vi "英维克通讯.vi"() -> ()   [LabVIEW 2016, in "环境动力监测库.lvlib" / "空调库.lvlib"]
uses:
  <vilib>/Plasmionique/MB Master/MB_Master/MB_Master.lvclass
  <vilib>/Plasmionique/MB Master/MB Master.lvlib
panel:
  out "遥控开关机状态":bool
  out "系统参数":T1
  out "告警状态":T2
  out "传感器状态":T3
  out "运行状态":T4
  out "遥控参数":u16[](array[numeric])
  out "系统参数":u16[](array[numeric])
  out "告警状态":u16[](array[numeric])
  out "传感器状态":u16[](array[numeric])
  out "运行状态":u16[](array[numeric])
  in  "读取数据":bool
  in  "释放串口":bool
  in  "打开串口":bool
  out "通讯状态":bool
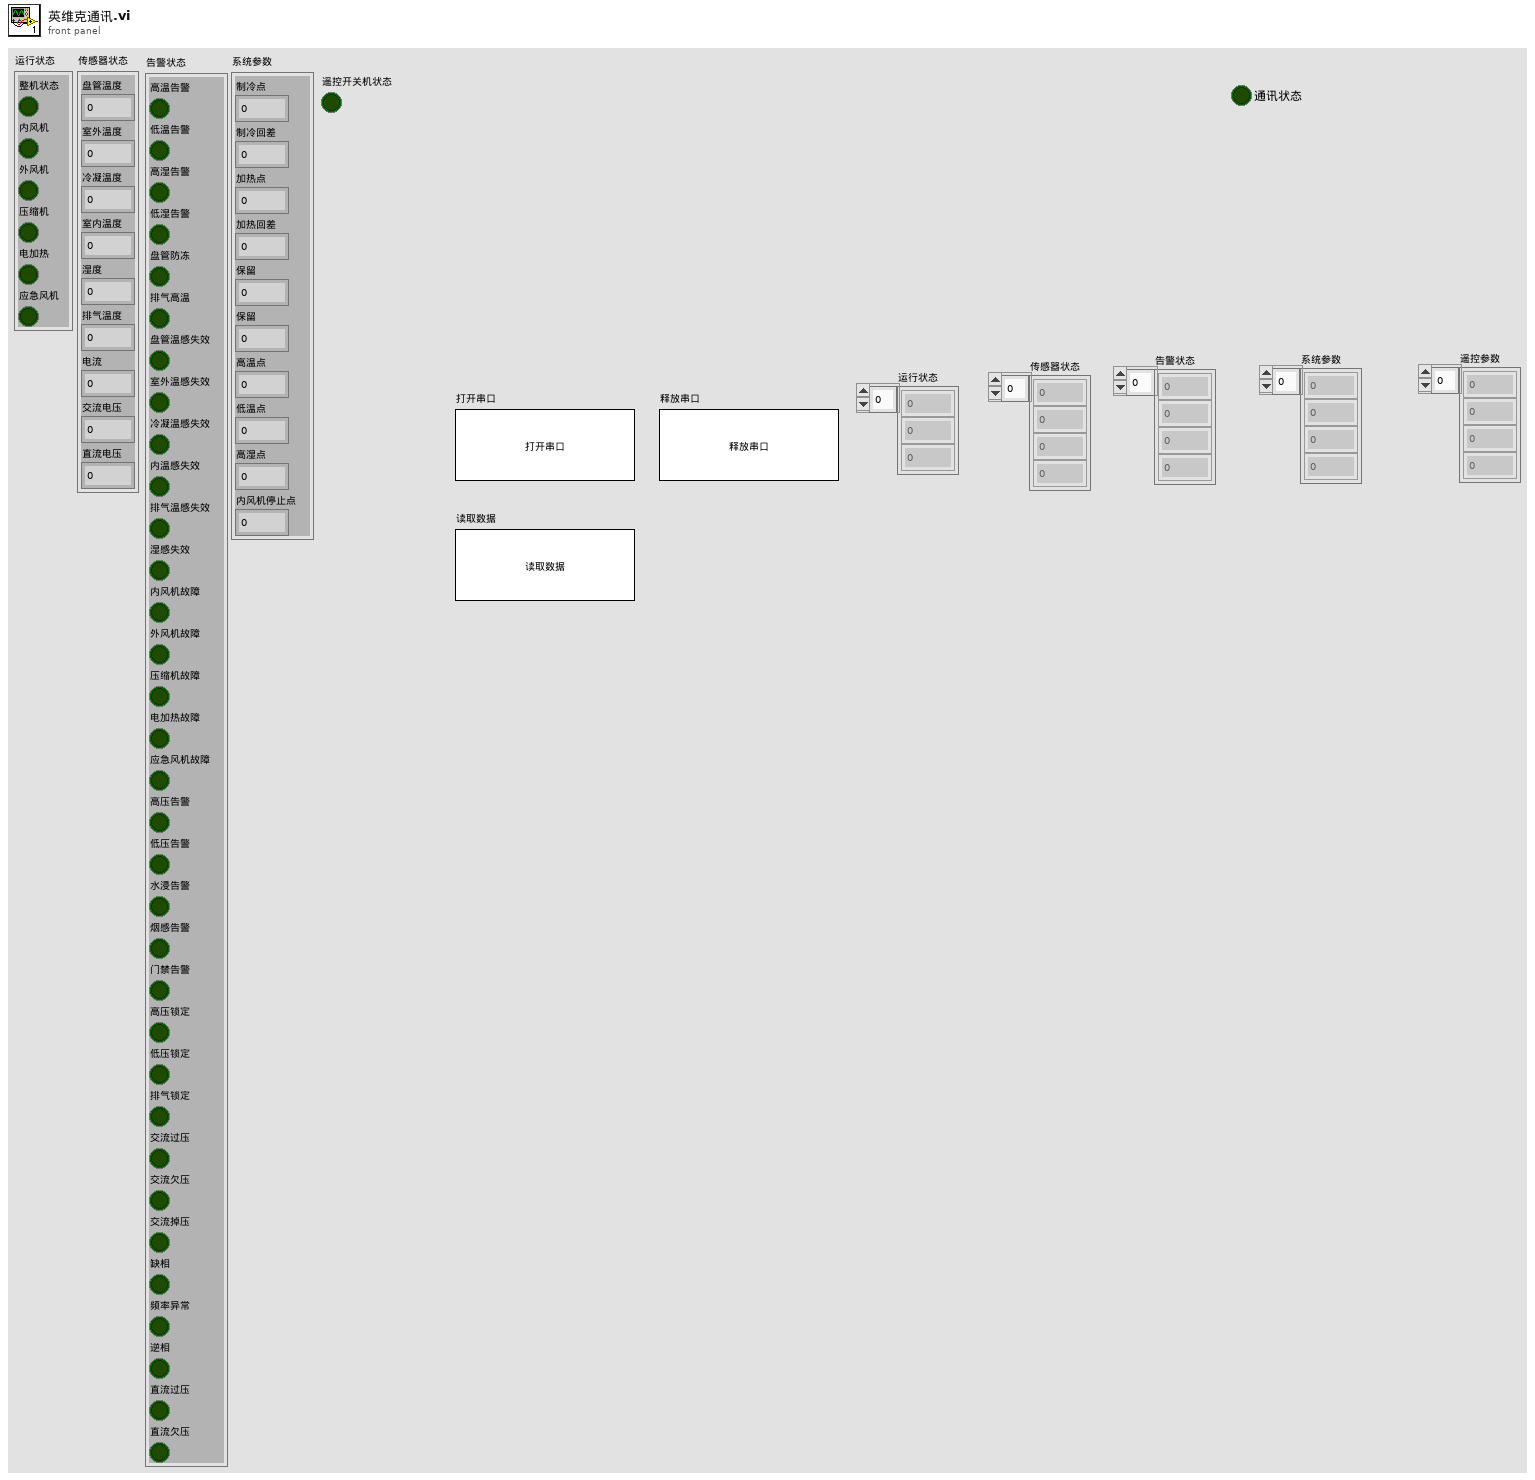
[diagram p1: front panel]
types:
  T1 = cluster{"制冷点":u16, "制冷回差":u16, "加热点":u16, "加热回差":u16, "保留":u16, "保留":u16, "高温点":u16, "低温点":u16, "高湿点":u16, "内风机停止点":u16}
  T2 = cluster{"高温告警":bool, "低温告警":bool, "高湿告警":bool, "低湿告警":bool, "盘管防冻":bool, "排气高温":bool, "盘管温感失效":bool, "室外温感失效":bool, "冷凝温感失效":bool, "内温感失效":bool, "排气温感失效":bool, "湿感失效":bool, "内风机故障":bool, "外风机故障":bool, "压缩机故障":bool, "电加热故障":bool, "应急风机故障":bool, "高压告警":bool, "低压告警":bool, "水浸告警":bool, "烟感告警":bool, "门禁告警":bool, "高压锁定":bool, "低压锁定":bool, "排气锁定":bool, "交流过压":bool, "交流欠压":bool, "交流掉压":bool, "缺相":bool, "频率异常":bool, "逆相":bool, "直流过压":bool, "直流欠压":bool}
  T3 = cluster{"盘管温度":u16, "室外温度":u16, "冷凝温度":u16, "室内温度":u16, "湿度":u16, "排气温度":u16, "电流":u16, "交流电压":u16, "直流电压":u16}
  T4 = cluster{"整机状态":bool, "内风机":bool, "外风机":bool, "压缩机":bool, "电加热":bool, "应急风机":bool}
  T5 = cluster{"型号选择":enum16{"黑盾", "英维克", "仁科测控RS-KTC-N01"}, "MB session in":refnum<class "MB_Master.lvclass">, "英维克空调寄存器":u16[], "通讯状态":bool, "PORT":string, "IP":string, "Slave ID ":u8, "Serial Config":cluster{"baud rate (bps)":u32, "stop bits":u16, "parity":u16, "flow control":u16, "timeout":u32, "retries":i32}, "VISA Resource":refnum<visa-resource-name>, "MB通信方式选择":enum16{"串口", "TCP"}, "系统参数":cluster{"空调开启点":u16, "空调灵敏点":u16, "加热开启点":u16, "加热灵敏度":u16, "高温告警点":u16, "低温告警点":u16}}
  T6 = enum16{"open", "read", "write single", "write", "close"}
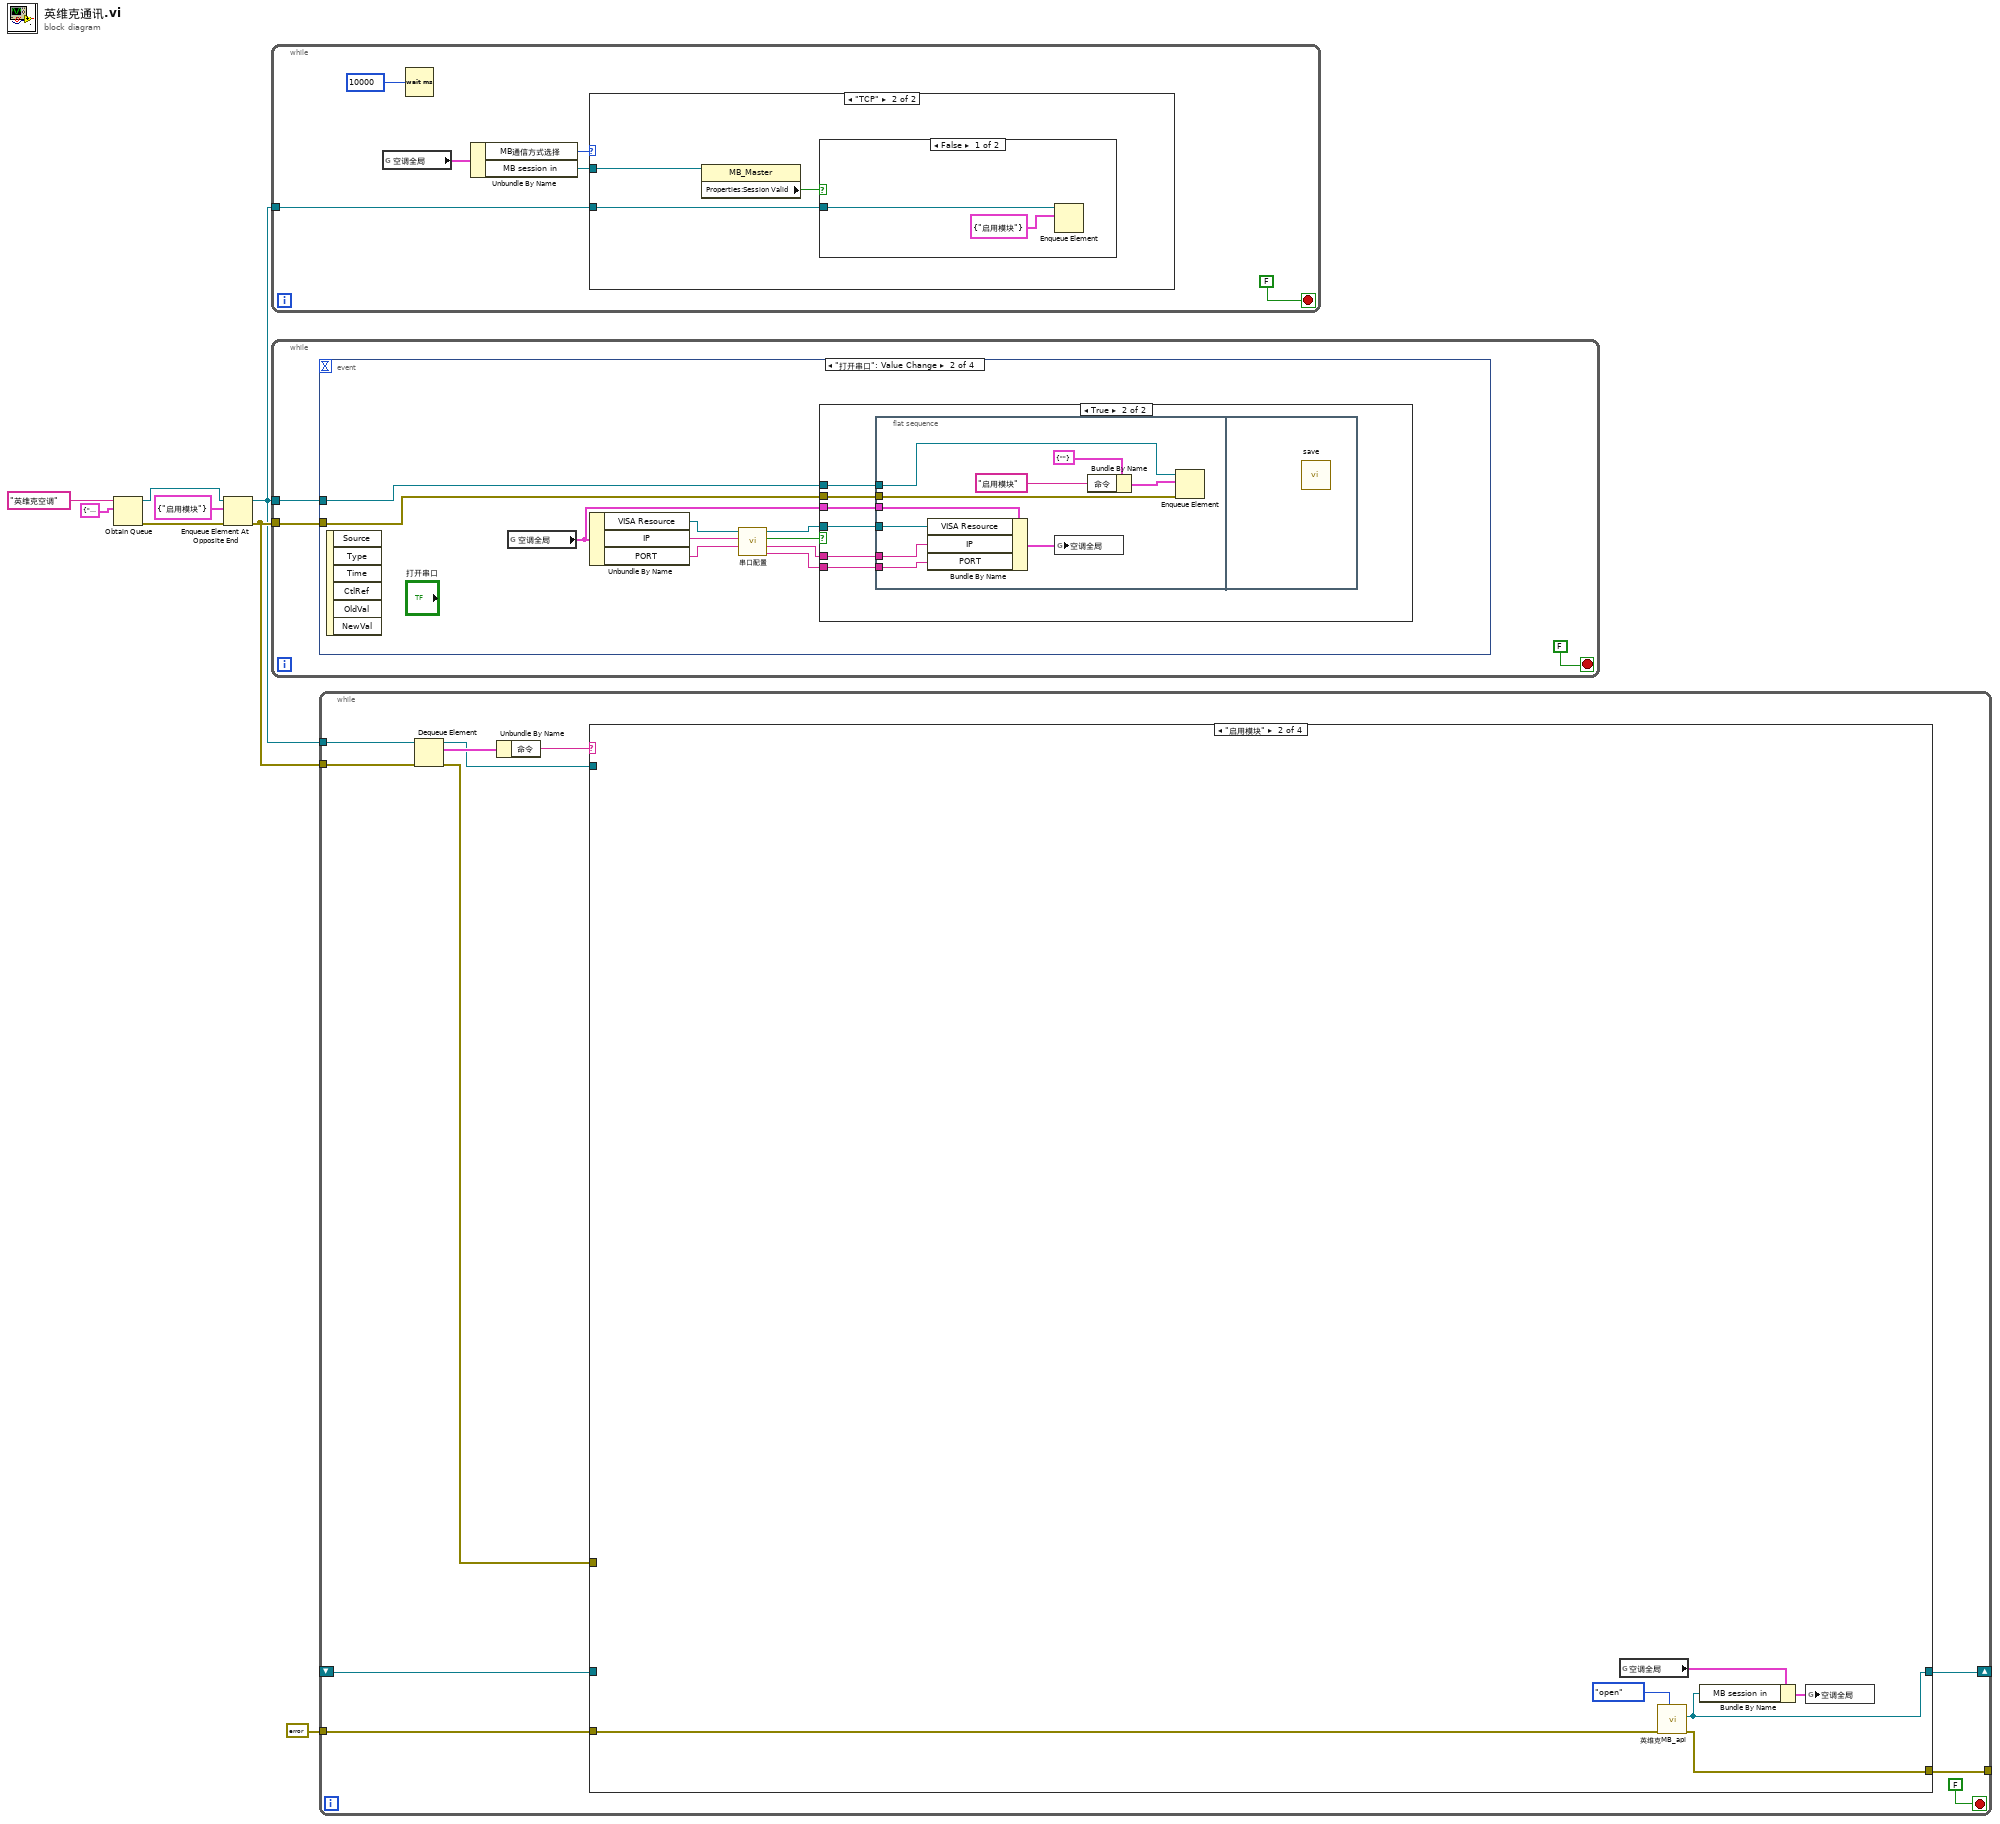
[diagram p0: block diagram]
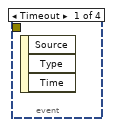
[diagram p4: hidden frame]
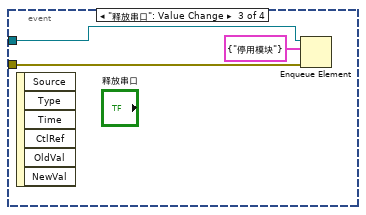
[diagram p6: hidden frame]
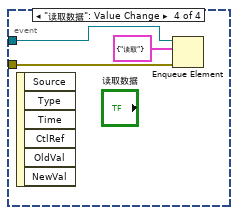
[diagram p7: hidden frame]
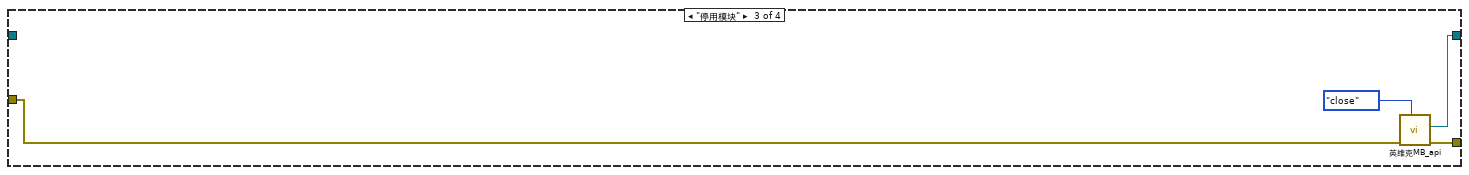
[diagram p9: hidden frame]
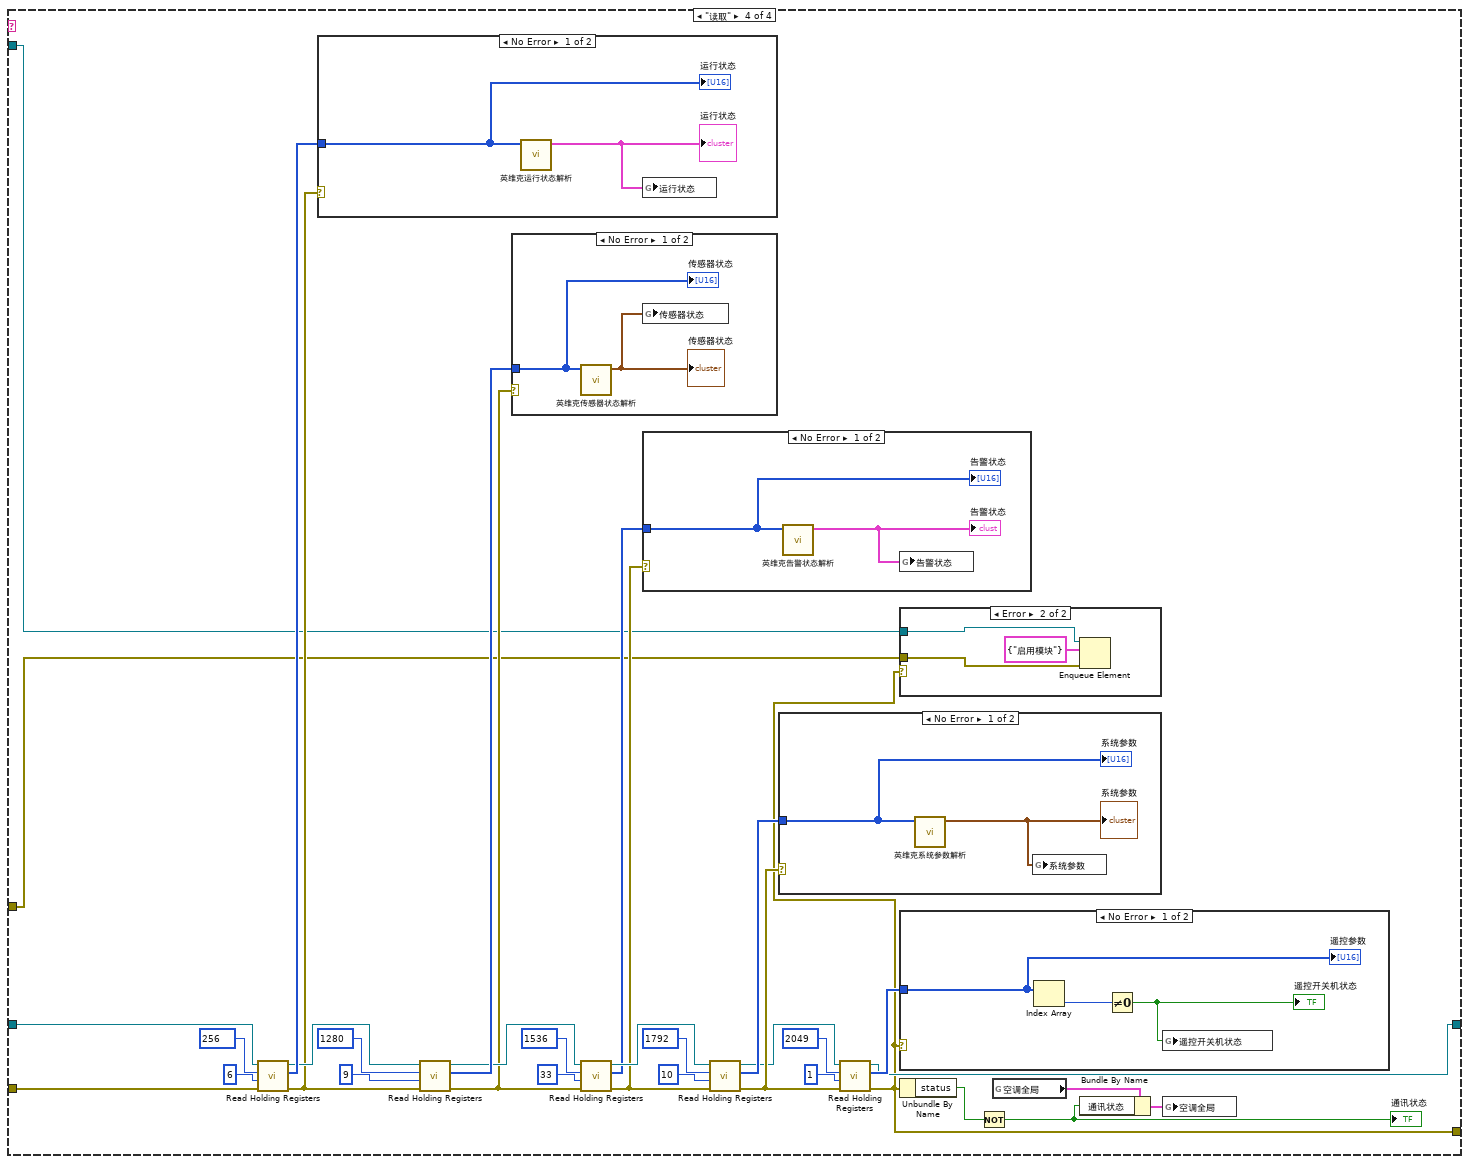
[diagram p10: hidden frame]
diagram:
  n1 = Obtain Queue(name (unnamed)="英维克空调" ("名称（未命名）"), element data type=cluster{"命令":string} {"命令"="启用模块"} ("元素")) -> (queue out=w5:refnum<queue>, error out=w4:errorcluster)  [unwired: 3 in, 1 out]
  n2 = Enqueue Element At Opposite End(queue=w5, element=cluster{"命令":string} {"命令"="启用模块"} ("元素"), error in (no error)=w4) -> (queue out=w1:refnum<queue>, error out=w2:errorcluster)  [unwired: 1 in, 1 out]
  n3 = while {
    tunnel: w1 -> [w14]
    stop <- FALSE stop-if-true
    n4 = global read "断电保存全局变量.vi" "空调全局"() -> (w11:T5)
    n5 = Wait (ms)(milliseconds to wait=u32 10000 ("等待时间（毫秒）")) -> ()  [unwired: 1 out]
    n6 = Unbundle By Name(w11) -> ("MB通信方式选择"=w10:enum16{"串口", "TCP"}, "MB session in"=w9:refnum<class "MB_Master.lvclass">)
    n7 = case shown="\"TCP\"" w10 {
      tunnel: w14 -> [_ w16]
      tunnel: w9 -> [_ w15]
      frame "串口", Default {
      }
      frame "TCP" {
        n8 = property class="MB_Master"(reference=w15) -> ("Properties:Session Valid"=w17:bool)  [unwired: 1 in, 2 out]
        n9 = case shown="False" w17 {
          tunnel: w16 -> [w19 _]
          frame False {
            n10 = Enqueue Element(queue=w19, element=cluster{"命令":string} {"命令"="启用模块"} ("元素")) -> ()  [unwired: 2 in, 3 out]
          }
          frame True {
          }
        }
      }
    }
  }
  n11 = while {
    tunnel: w1 -> [w21]
    tunnel: w2 -> [w20]
    stop <- FALSE stop-if-true
    n12 = event shown="[1] \"打开串口\": Value Change" {
      selector: _ -> [_ _ _ _]
      dyn-events: _ -> [_ _ _ _]
      timeout: _ -> [_ _ _ _]
      tunnel: w21 -> [_ w32 w51 w53]
      tunnel: w20 -> [_ w31 w50 w52]
      event Timeout {
        n13 = event-data() -> ()  [unwired: 1 in, 3 out]
      }
      event "打开串口": Value Change {
        n14 = event-data() -> ()  [unwired: 1 in, 6 out]
        n15 = global read "断电保存全局变量.vi" "空调全局"() -> (w23:T5)
        n16 = Unbundle By Name(w23) -> ("VISA Resource"=w26:refnum<visa-resource-name>, "IP"=w25:string, "PORT"=w24:string)
        n17 = call "串口配置.vi"("PORT"=w24, "IP"=w25, "请选择串口:"=w26) -> ("PORT 2"=w27:string, "IP 2"=w28:string, "确认 2"=w29:bool, "VISA资源名称 2"=w30:refnum<visa-resource-name>)  [unwired: 5 in]
        n18 = case shown="True" w29 {
          tunnel: w30 -> [_ w36]
          tunnel: w32 -> [_ w38]
          tunnel: w31 -> [_ w37]
          tunnel: w28 -> [_ w35]
          tunnel: w27 -> [_ w34]
          tunnel: w23 -> [_ w33]
          frame False {
          }
          frame True {
            n19 = flat-sequence {
              tunnel: w38 -> [w45]
              tunnel: w37 -> [w44]
              tunnel: w36 -> [w41]
              tunnel: w35 -> [w40]
              tunnel: w34 -> [w39]
              tunnel: w33 -> [w43]
              frame #0 {
                n20 = Bundle By Name(cluster=w43, "VISA Resource"=w41, "IP"=w40, "PORT"=w39) -> (w42:T5)
                n21 = global write "断电保存全局变量.vi" "空调全局"(w42) -> ()
                n22 = Bundle By Name(cluster=cluster{"命令":string} {"命令"=""} ("元素"), "命令"="启用模块" ("名称（未命名）")) -> (w46:cluster{"命令":string})
                n23 = Enqueue Element(queue=w45, element=w46, error in (no error)=w44) -> ()  [unwired: 1 in, 3 out]
              }
              frame #1 {
                n24 = call "save.vi"() -> ()  [unwired: 11 in, 1 out]
              }
            }
          }
        }
      }
      event "释放串口": Value Change {
        n25 = event-data() -> ()  [unwired: 1 in, 6 out]
        n26 = Enqueue Element(queue=w51, element=cluster{"命令":string} {"命令"="停用模块"} ("元素"), error in (no error)=w50) -> ()  [unwired: 1 in, 3 out]
      }
      event "读取数据": Value Change {
        n27 = event-data() -> ()  [unwired: 1 in, 6 out]
        n28 = Enqueue Element(queue=w53, element=cluster{"命令":string} {"命令"="读取"} ("元素"), error in (no error)=w52) -> ()  [unwired: 1 in, 3 out]
      }
    }
  }
  n29 = while {
    tunnel: w1 -> [w57]
    tunnel: w2 -> [w64]
    tunnel: [w58] -> _
    shift-right: [w61] -> _
    shift-left: _ -> [w60]
    tunnel: errorcluster {"status"=FALSE, "code"=0, "source"=""} ("error out") -> [w59]
    stop <- FALSE stop-if-true
    n30 = Dequeue Element(queue=w57, error in (no error)=w64) -> (queue out=w56:refnum<queue>, element=w63:cluster{"命令":string}, error out=w55:errorcluster)  [unwired: 1 in, 1 out]
    n31 = Unbundle By Name(w63) -> ("命令"=w62:string)
    n32 = case shown="\"启用模块\"" w62 {
      tunnel: [w67 w68 w75 w84] -> w61
      tunnel: [w66 w73 w76 w81] -> w58
      tunnel: w60 -> [w67 _ _ w110]
      tunnel: w59 -> [w66 w72 w77 w109]
      tunnel: w56 -> [_ _ _ w83]
      tunnel: w55 -> [_ _ _ w82]
      frame Default {
      }
      frame "启用模块" {
        n33 = global read "断电保存全局变量.vi" "空调全局"() -> (w70:T5)
        n34 = call "英维克MB_api.vi"("STEP"=T6."open", "Error in"=w72) -> ("error out"=w73:errorcluster, "MB session out"=w68:refnum<class "MB_Master.lvclass">)  [unwired: 7 in, 1 out]
        n35 = Bundle By Name(cluster=w70, "MB session in"=w68) -> (w69:T5)
        n36 = global write "断电保存全局变量.vi" "空调全局"(w69) -> ()
      }
      frame "停用模块" {
        n37 = call "英维克MB_api.vi"("STEP"=T6."close", "Error in"=w77) -> ("error out"=w76:errorcluster, "MB session out"=w75:refnum<class "MB_Master.lvclass">)  [unwired: 7 in, 1 out]
      }
      frame "读取" {
        n38 = call <vilib>:"Read Holding Registers.vi"("error in (no error)"=w109, "quantity"=u16 6 ("number of holding registers"), "starting address"=u16 256, "MB session in"=w110) -> ("error out"=w106:errorcluster, "Registers"=w108:u16[], "MB session out"=w107:refnum<class "MB_Master.lvclass">)  [unwired: 5 in]
        n39 = case shown="No Error" w106 {
          tunnel: w108 -> [w124 _]
          frame No Error {
            n40 = call "英维克运行状态解析.vi"("运行状态输入"=w124) -> ("运行状态"=w123:T4)  [unwired: 10 in]
            "运行状态" <- w123
            n41 = global write "内部交互全局变量.vi" "运行状态"(w123) -> ()
            "运行状态" <- w124
          }
          frame Error {
          }
        }
        n42 = call <vilib>:"Read Holding Registers.vi"("error in (no error)"=w106, "quantity"=u16 9 ("number of holding registers"), "starting address"=u16 1280, "MB session in"=w107) -> ("error out"=w98:errorcluster, "Registers"=w105:u16[], "MB session out"=w99:refnum<class "MB_Master.lvclass">)  [unwired: 5 in]
        n43 = case shown="No Error" w98 {
          tunnel: w105 -> [w122 _]
          frame No Error {
            n44 = call "英维克传感器状态解析.vi"("传感器状态输入"=w122) -> ("传感器状态输出"=w121:T3)  [unwired: 10 in]
            "传感器状态" <- w121
            n45 = global write "内部交互全局变量.vi" "传感器状态"(w121) -> ()
            "传感器状态" <- w122
          }
          frame Error {
          }
        }
        n46 = call <vilib>:"Read Holding Registers.vi"("error in (no error)"=w98, "quantity"=u16 33 ("number of holding registers"), "starting address"=u16 1536, "MB session in"=w99) -> ("error out"=w92:errorcluster, "Registers"=w91:u16[], "MB session out"=w93:refnum<class "MB_Master.lvclass">)  [unwired: 5 in]
        n47 = case shown="No Error" w92 {
          tunnel: w91 -> [w120 _]
          frame No Error {
            n48 = call "英维克告警状态解析.vi"("告警状态输入"=w120) -> ("告警状态"=w119:T2)  [unwired: 10 in]
            "告警状态" <- w119
            n49 = global write "内部交互全局变量.vi" "告警状态"(w119) -> ()
            "告警状态" <- w120
          }
          frame Error {
          }
        }
        n50 = call <vilib>:"Read Holding Registers.vi"("error in (no error)"=w92, "quantity"=u16 10 ("number of holding registers"), "starting address"=u16 1792, "MB session in"=w93) -> ("error out"=w87:errorcluster, "Registers"=w90:u16[], "MB session out"=w86:refnum<class "MB_Master.lvclass">)  [unwired: 5 in]
        n51 = case shown="No Error" w87 {
          tunnel: w90 -> [w118 _]
          frame No Error {
            n52 = call "英维克系统参数解析.vi"("系统参数输入"=w118) -> ("系统参数"=w117:T1)  [unwired: 10 in]
            "系统参数" <- w117
            n53 = global write "内部交互全局变量.vi" "系统参数"(w117) -> ()
            "系统参数" <- w118
          }
          frame Error {
          }
        }
        n54 = call <vilib>:"Read Holding Registers.vi"("error in (no error)"=w87, "quantity"=u16 1 ("number of holding registers"), "starting address"=u16 2049, "MB session in"=w86) -> ("error out"=w81:errorcluster, "Registers"=w85:u16[], "MB session out"=w84:refnum<class "MB_Master.lvclass">)  [unwired: 5 in]
        n55 = case shown="Error" w81 {
          tunnel: w83 -> [_ w113]
          tunnel: w82 -> [_ w111]
          frame No Error {
          }
          frame Error {
            n56 = Enqueue Element(queue=w113, element=cluster{"命令":string} {"命令"="启用模块"} ("元素"), error in (no error)=w111) -> ()  [unwired: 1 in, 3 out]
          }
        }
        n57 = case shown="No Error" w81 {
          tunnel: w85 -> [w116 _]
          frame No Error {
            n58 = Index Array(array=w116) -> (element=w115:u16)  [unwired: 1 in]
            n59 = Not Equal To 0?(x=w115) -> (x != 0?=w114:bool)
            "遥控开关机状态" <- w114
            n60 = global write "内部交互全局变量.vi" "遥控开关机状态"(w114) -> ()
            "遥控参数" <- w116
          }
          frame Error {
          }
        }
        n61 = Unbundle By Name(w81) -> ("status"=w100:bool)
        n62 = Not(x=w100) -> (.not. x?=w79:bool)
        "通讯状态" <- w79
        n63 = global read "断电保存全局变量.vi" "空调全局"() -> (w80:T5)
        n64 = Bundle By Name(cluster=w80, "通讯状态"=w79) -> (w78:T5)
        n65 = global write "断电保存全局变量.vi" "空调全局"(w78) -> ()
      }
    }
  }
